vi "VelSimpleEstBall.vi"(7 "dt":dbl, 10 "Balls Out":T1[](array[typedef]), 11 "Balls Out 2":T1[](array[typedef])) -> (3 "Array":T1[](array[typedef]))   [LabVIEW 2018]
uses:
  SSL Detection Ball.ctl
  <vilib>/Analysis/Matrix/Datatypes/RealMatrix.ctl
  <vilib>/Analysis/Matrix/NI_Matrix.lvlib
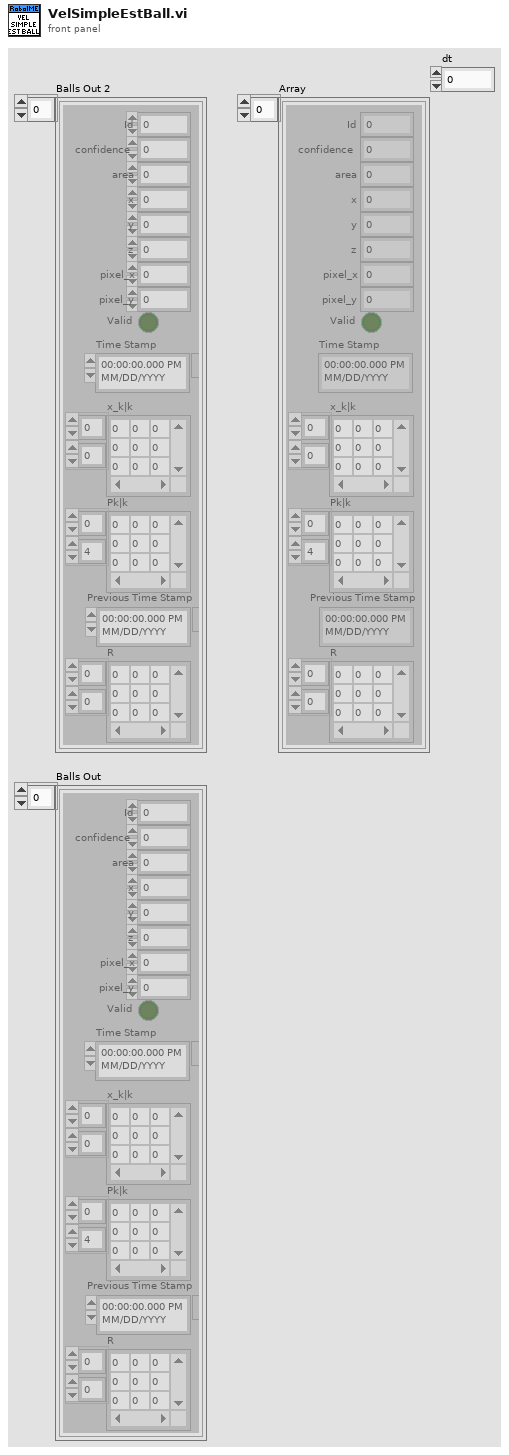
[diagram p1: front panel]
types:
  T1 = typedef "SSL Detection Ball.ctl" = cluster{"x":sgl, "area":u32, "confidence":sgl, "y":sgl, "z":sgl, "pixel_x":sgl, "pixel_y":sgl, "Valid":bool, "Time Stamp":timestamp, "x_k|k":T2, "Pk|k":T2, "Id":u32, "Previous Time Stamp":timestamp, "R":T2}
  T2 = typedef "NI_Matrix.lvlib/RealMatrix.ctl" = dbl[][]
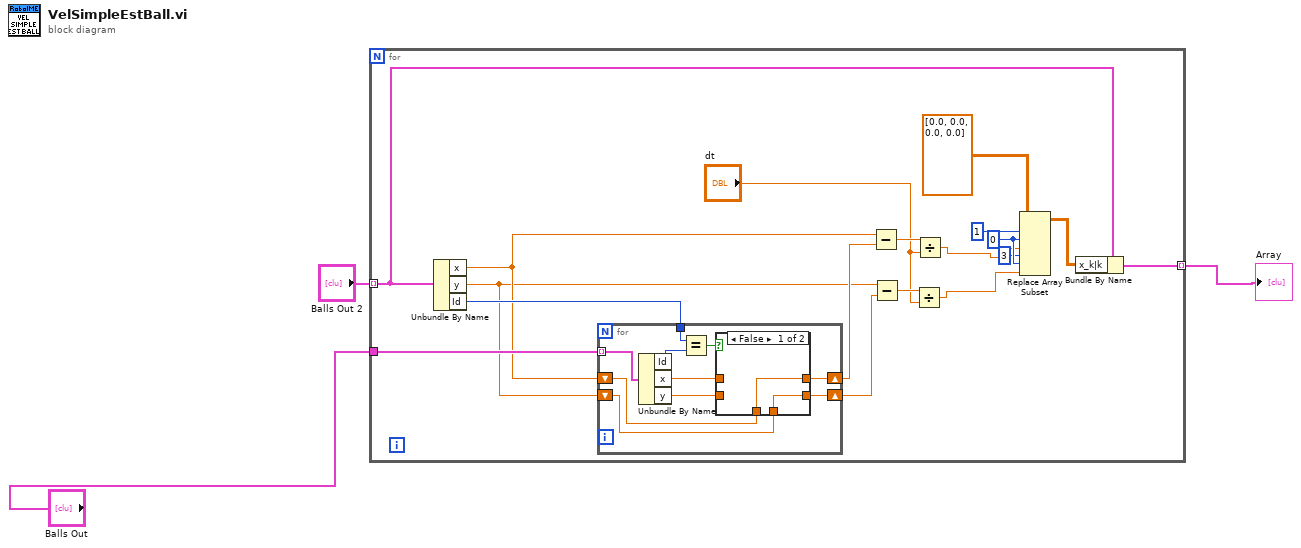
[diagram p0: block diagram]
diagram:
  n1 = for {
    tunnel: "Balls Out 2" -> [w13] mode=indexing
    tunnel: "Balls Out" -> [w21]
    tunnel: [w12] -> w3 mode=indexing
    w9 = 0 ("disabled index (col)")
    n2 = Unbundle By Name(w13) -> ("x"=w19:sgl, "y"=w17:sgl, "Id"=w20:u32)
    n3 = for {
      tunnel: w21 -> [w31] mode=indexing
      tunnel: w20 -> [w28]
      shift-right: [w27] -> w18
      shift-left: w19 -> [w23]
      shift-right: [w24] -> w16
      shift-left: w17 -> [w22]
      n4 = Unbundle By Name(w31) -> ("Id"=w29:u32, "x"=w26:sgl, "y"=w25:sgl)
      n5 = Equal?(x=w28, y=w29) -> (x = y?=w30:bool)
      n6 = case shown="False" w30 {
        tunnel: [w33 w35] -> w27
        tunnel: w26 -> [_ w35]
        tunnel: [w32 w34] -> w24
        tunnel: w25 -> [_ w34]
        tunnel: w23 -> [w33 _]
        tunnel: w22 -> [w32 _]
        frame False {
        }
        frame True {
        }
      }
    }
    n7 = Subtract(x=w19, y=w18) -> (x-y=w15:sgl)
    n8 = Subtract(x=w17, y=w16) -> (x-y=w14:sgl)
    n9 = Divide(x=w14, y="dt") -> (x/y=w5:dbl)
    n10 = Divide(x=w15, y="dt") -> (x/y=w6:dbl)
    n11 = Replace Array Subset(array=T2 [[0.0], [0.0], [0.0], [0.0]] ("x_k|k"), new element #1=w6, index (row) #1=1 ("index (row)"), index (col) #1=w9, new element #2=w5, index (row) #2=3 ("disabled index (row)"), index (col) #2=w9) -> (w7:T2)
    n12 = Bundle By Name(cluster=w13, "x_k|k"=w7) -> (w12:T1)
  }
  "Array" <- w3
